vi "libssh2_userauth_authenticated.vi"(8 "error in (no error)":errorcluster, 11 "session":T1) -> (0 "error out":errorcluster, 2 "authenticated":bool)   [LabVIEW 2013, in "libssh2.lvlib"]
doc: "Get a value indicating if a session has been authenticated."
uses:
  libssh2.lvlib
  Session Refnum.ctl
  Not A Session.vi
  <vilib>/Utility/error.llb/Error Cluster From Error Code.vi
  Global Settings.vi
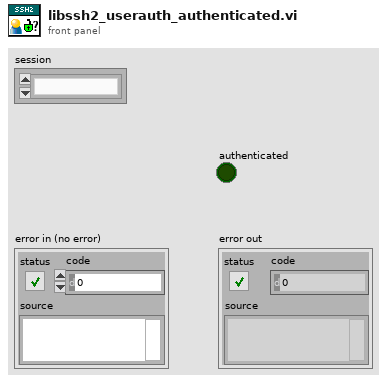
[diagram p1: front panel]
types:
  T1 = typedef "libssh2.lvlib/Session Refnum.ctl" = refnum<k1>
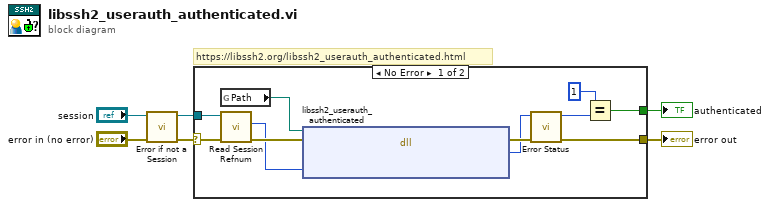
[diagram p0: block diagram]
diagram:
  # "https://libssh2.org/libssh2_userauth_authenticated.html"
  n1 = call "Error if not a Session.vi"("error in (no error)"="error in (no error)", "session"="session") -> ("error out"=w3:errorcluster, "session out"=w1:T1)  [unwired: 8 in]
  n2 = case shown="No Error" w3 {
    selector: w3 -> [w14 w18]
    tunnel: [w11 w18] -> w6
    tunnel: [w8 _] -> w5
    tunnel: w1 -> [w16 _]
    frame No Error {
      n3 = global read "Global Settings.vi" "Path"() -> (w12:path)
      n4 = call "Read Session Refnum.vi"("error in (no error)"=w14, "session"=w16) -> ("error out"=w17:errorcluster, "LIBSSH2_SESSION*"=w15:u64)  [unwired: 5 in, 3 out]
      n5 = dll-call lib="?" fn="libssh2_userauth_authenticated"(path in=w12, error in=w17, "session"=w15) -> (error out=w13:errorcluster, "return value"=w10:i32)  [unwired: 2 in, 1 out]
      n6 = call "Error Status.vi"("error in (no error)"=w13, "return value"=w10) -> ("error out"=w11:errorcluster, "return value out"=w9:i32)  [unwired: 8 in]
      n7 = Equal?(x=1, y=w9) -> (x = y?=w8:bool)
    }
    frame Error {
    }
  }
  "error out" <- w6
  "authenticated" <- w5
